vi "Test Joystick.vi"() -> ()   [LabVIEW 2018]
uses:
  <vilib>/Instr/_visa.llb/VISA Configure Serial Port (Instr).vi
panel:
  in  "TITL":bool
  in  "PAN":bool
  out "pan":dbl
  out "tilt angle":dbl format="%.2f"
  in  "autoFocus":bool
  out "Cam rcv":string
  in  "Clear":bool
  in  "Menu":bool caption="Open"
  in  "Aux":bool caption="Open"
  in  "Tele":bool caption="Open"
  in  "wide":bool caption="Wide"
  in  "OFF":bool caption="Open"
  in  "ON":bool caption="Open"
  in  "Near":bool caption="Open"
  in  "Far":bool
  in  "ACK":bool caption="Open"
  in  "Shot":bool caption="Open"
  in  "Open":bool
  in  "Close":bool
  out "Keypad sent":string
  in  "VISA resource name 2":refnum<visa-resource-name>
  in  "Stop Button":bool
  in  "VISA resource name":refnum<visa-resource-name>
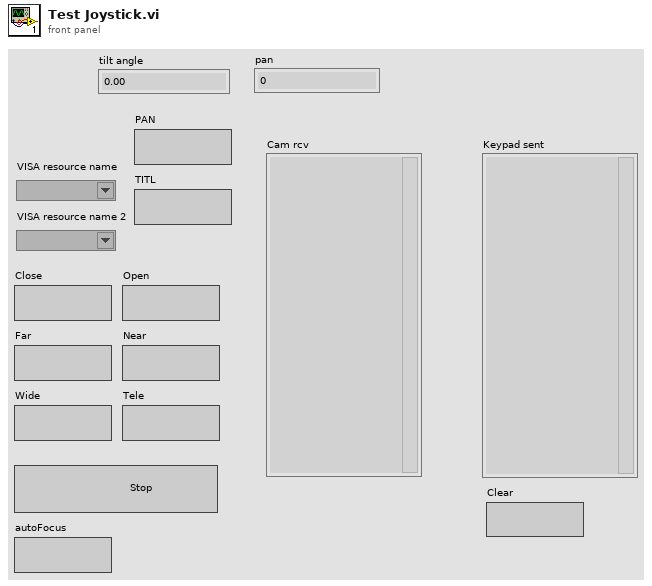
[diagram p1: front panel]
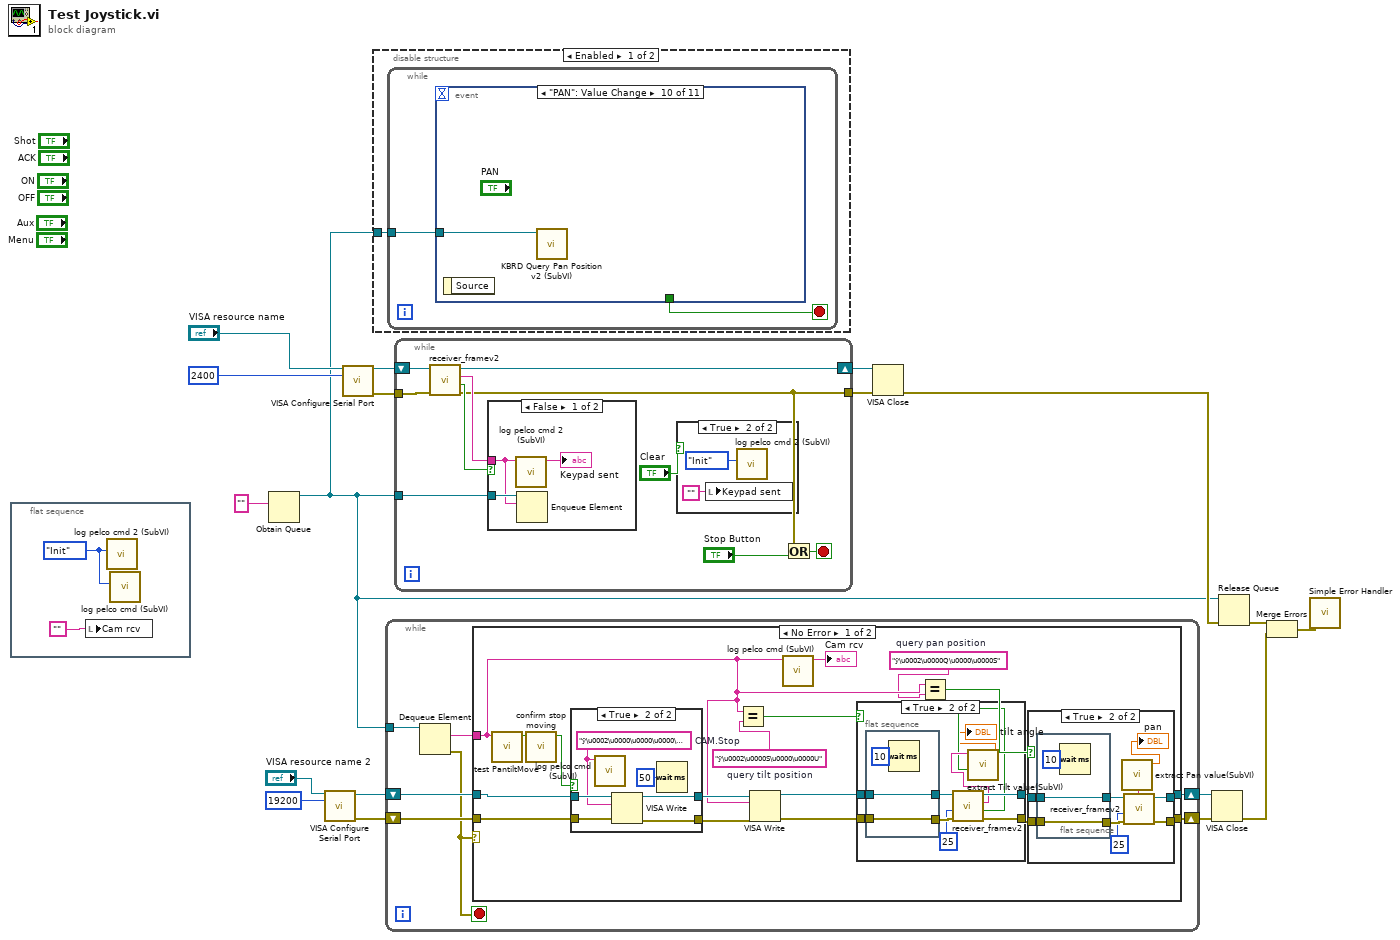
[diagram p0: block diagram]
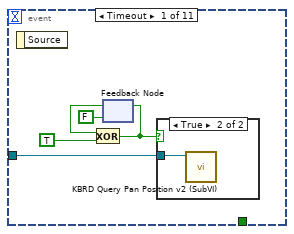
[diagram p2: hidden frame]
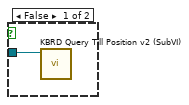
[diagram p3: hidden frame]
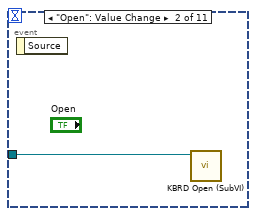
[diagram p4: hidden frame]
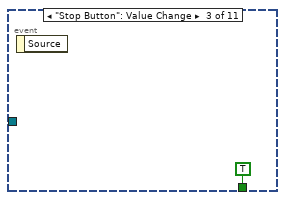
[diagram p5: hidden frame]
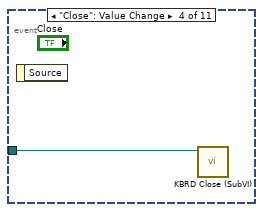
[diagram p6: hidden frame]
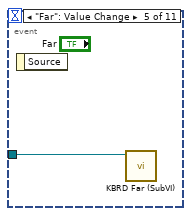
[diagram p7: hidden frame]
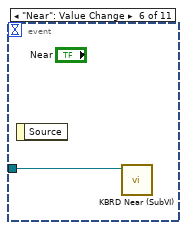
[diagram p8: hidden frame]
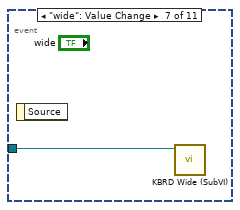
[diagram p9: hidden frame]
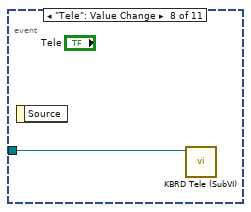
[diagram p10: hidden frame]
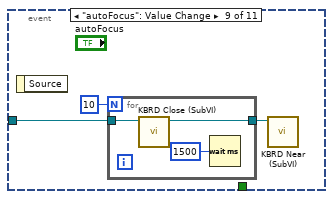
[diagram p11: hidden frame]
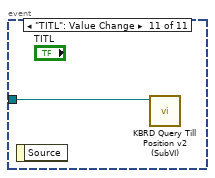
[diagram p12: hidden frame]
diagram:
  n1 = flat-sequence {
    frame #0 {
      w20 = enum16{"Log", "Init"}."Init" ("Enum(log)")
      n2 = local write "Cam rcv"("") -> ()
      n3 = call "log pelco cmd 2 (SubVI).vi"("Enum(log)"=w20) -> ()  [unwired: 10 in, 1 out]
      n4 = call "log pelco cmd (SubVI).vi"("Enum(log)"=w20) -> ()  [unwired: 10 in, 1 out]
    }
  }
  n5 = Obtain Queue(element data type="") -> (queue out=w1:refnum<queue>)  [unwired: 4 in, 2 out]
  n6 = call-poly "VISA Configure Serial Port"("VISA resource name"="VISA resource name 2", "baud rate (9600)"=u32 19200) -> ("VISA resource name out"=w9:refnum<visa-resource-name>, "error out"=w8:errorcluster)  [unwired: 12 in]
  n7 = call-poly "VISA Configure Serial Port"("VISA resource name"="VISA resource name", "baud rate (9600)"=u32 2400) -> ("VISA resource name out"=w16:refnum<visa-resource-name>, "error out"=w15:errorcluster)  [unwired: 12 in]
  n8 = disable-structure shown="Enabled" {
    disable-tunnel: w1 -> [w21 _]
    frame Enabled {
      n9 = while {
        tunnel: w21 -> [w23]
        stop <- w22 stop-if-true
        n10 = event shown="[9] \"PAN\": Value Change" {
          selector: _ -> [_ _ _ _ _ _ _ _ _ _ _]
          dyn-events: _ -> [_ _ _ _ _ _ _ _ _ _ _]
          timeout: _ -> [_ _ _ _ _ _ _ _ _ _ _]
          tunnel: w23 -> [w24 w31 _ w33 w34 w35 w36 w37 w39 w44 w45]
          tunnel: [_ _ TRUE _ _ _ _ _ _ _ _] -> w22
          event Timeout {
            n11 = event-data() -> ()  [unwired: 1 in, 1 out]
            n12 = feedback #1(FALSE) -> (w27:bool)
            n13 = Exclusive Or(1:TRUE, 2:w27) -> (0:w26:bool)
            n14 = feedback-in #1(w26) -> ()
            n15 = case shown="True" w26 {
              tunnel: w24 -> [w29 w30]
              frame False {
                n16 = call "KBRD Query Till Position v2 (SubVI).vi"("Queue in"=w29) -> ()  [unwired: 10 in, 1 out]
              }
              frame True {
                n17 = call "KBRD Query Pan Position v2 (SubVI).vi"("Queue in"=w30) -> ()  [unwired: 10 in, 1 out]
              }
            }
          }
          event "Open": Value Change {
            n18 = event-data() -> ()  [unwired: 1 in, 1 out]
            n19 = call "KBRD Open (SubVI).vi"("Queue in"=w31) -> ()  [unwired: 11 in]
          }
          event "Stop Button": Value Change {
            n20 = event-data() -> ()  [unwired: 1 in, 1 out]
          }
          event "Close": Value Change {
            n21 = event-data() -> ()  [unwired: 1 in, 1 out]
            n22 = call "KBRD Close (SubVI).vi"("Queue in"=w33) -> ()  [unwired: 10 in, 1 out]
          }
          event "Far": Value Change {
            n23 = event-data() -> ()  [unwired: 1 in, 1 out]
            n24 = call "KBRD Far (SubVI).vi"("Queue in"=w34) -> ()  [unwired: 11 in]
          }
          event "Near": Value Change {
            n25 = event-data() -> ()  [unwired: 1 in, 1 out]
            n26 = call "KBRD Near (SubVI).vi"("Queue in"=w35) -> ()  [unwired: 11 in]
          }
          event "wide": Value Change {
            n27 = event-data() -> ()  [unwired: 1 in, 1 out]
            n28 = call "KBRD Wide (SubVI).vi"("Queue in"=w36) -> ()  [unwired: 11 in]
          }
          event "Tele": Value Change {
            n29 = event-data() -> ()  [unwired: 1 in, 1 out]
            n30 = call "KBRD Tele (SubVI).vi"("Queue in"=w37) -> ()  [unwired: 11 in]
          }
          event "autoFocus": Value Change {
            n31 = event-data() -> ()  [unwired: 1 in, 1 out]
            n32 = for {
              N: 10 -> [_]
              tunnel: w39 -> [w43]
              tunnel: [w42] -> w38
              n33 = call "KBRD Close (SubVI).vi"("Queue in"=w43) -> ("dup Quece"=w42:refnum<queue>)  [unwired: 10 in]
              n34 = Wait (ms)(milliseconds to wait=u32 1500) -> ()  [unwired: 1 out]
            }
            n35 = call "KBRD Near (SubVI).vi"("Queue in"=w38) -> ()  [unwired: 11 in]
          }
          event "PAN": Value Change {
            n36 = event-data() -> ()  [unwired: 1 in, 1 out]
            n37 = call "KBRD Query Pan Position v2 (SubVI).vi"("Queue in"=w44) -> ()  [unwired: 10 in, 1 out]
          }
          event "TITL": Value Change {
            n38 = event-data() -> ()  [unwired: 1 in, 1 out]
            n39 = call "KBRD Query Till Position v2 (SubVI).vi"("Queue in"=w45) -> ()  [unwired: 10 in, 1 out]
          }
        }
      }
    }
    frame Disabled {
    }
  }
  n40 = while {
    tunnel: w1 -> [w52]
    shift-right: [w49] -> w7
    shift-left: w8 -> [w50]
    shift-right: [w47] -> w6
    shift-left: w9 -> [w51]
    stop <- w46 stop-if-true
    n41 = Dequeue Element(queue=w52) -> (element=w48:string, error out=w46:errorcluster)  [unwired: 2 in, 2 out]
    n42 = case shown="No Error" w46 {
      tunnel: w51 -> [w68 w110]
      tunnel: w50 -> [w67 w109]
      tunnel: [w53 w109] -> w49
      tunnel: w48 -> [w59 _]
      tunnel: [w54 w110] -> w47
      frame No Error {
        w58 = "ÿ\u0002\u0000Q\u0000\u0000S"  # query pan position
        w63 = "ÿ\u0002\u0000S\u0000\u0000U"  # query tilt position
        n43 = call "test PantiltMove.vi"("PelcoD frame"=w59) -> ("Pantilt Move?"=w70:bool)  [unwired: 10 in]
        n44 = call "confirm stop moving.vi"("moving?"=w70) -> ("Boolean"=w69:bool)  [unwired: 10 in]
        n45 = case shown="True" w69 {
          tunnel: w68 -> [w102 w108]
          tunnel: w67 -> [w101 w107]
          tunnel: [w101 w106] -> w66
          tunnel: [w102 w105] -> w65
          frame False {
          }
          frame True {
            w104 = "ÿ\u0002\u0000\u0000\u0000\u0000\u0002"  # CAM.Stop
            n46 = call "log pelco cmd (SubVI).vi"("String"=w104) -> ()  [unwired: 10 in, 1 out]
            n47 = VISA Write(VISA resource name=w108, write buffer=w104, error in (no error)=w107) -> (VISA resource name out=w105:refnum<visa-resource-name>, error out=w106:errorcluster)  [unwired: 1 out]
            n48 = Wait (ms)(milliseconds to wait=u32 50) -> ()  [unwired: 1 out]
          }
        }
        n49 = Equal?(x=w59, y=w63) -> (x = y?=w62:bool)
        n50 = VISA Write(VISA resource name=w65, write buffer=w59, error in (no error)=w66) -> (VISA resource name out=w61:refnum<visa-resource-name>, error out=w60:errorcluster)  [unwired: 1 out]
        n51 = call "log pelco cmd (SubVI).vi"("String"=w59) -> ("Cam rcv"=→"Cam rcv":string)  [unwired: 10 in]
        n52 = case shown="True" w62 {
          tunnel: w61 -> [w87 w97]
          tunnel: w60 -> [w86 w96]
          tunnel: [w87 w93] -> w56
          tunnel: [w86 w92] -> w55
          frame False {
          }
          frame True {
            n53 = flat-sequence {
              tunnel: [w99] -> w94
              tunnel: w97 -> [w99]
              tunnel: [w98] -> w95
              tunnel: w96 -> [w98]
              frame #0 {
                n54 = Wait (ms)(milliseconds to wait=u32 10) -> ()  [unwired: 1 out]
              }
            }
            n55 = call "receiver_framev2.vi"("error in (no error)"=w95, "Timeout(100ms)"=u32 25, "Visa In"=w94) -> ("error out"=w92:errorcluster, "TimeOut?"=w89:bool, "response"=w90:string, "Visa out"=w93:refnum<visa-resource-name>)  [unwired: 5 in]
            n56 = call "extract Tilt value(SubVI).vi"("Time out?"=w89, "Pelco-D response"=w90) -> ("tilt1"=→"tilt angle":dbl)  [unwired: 8 in, 1 out]
          }
        }
        n57 = Equal?(x=w59, y=w58) -> (x = y?=w57:bool)
        n58 = case shown="True" w57 {
          tunnel: w56 -> [w72 w82]
          tunnel: w55 -> [w71 w81]
          tunnel: [w72 w78] -> w54
          tunnel: [w71 w77] -> w53
          frame False {
          }
          frame True {
            n59 = flat-sequence {
              tunnel: [w84] -> w79
              tunnel: w82 -> [w84]
              tunnel: [w83] -> w80
              tunnel: w81 -> [w83]
              frame #0 {
                n60 = Wait (ms)(milliseconds to wait=u32 10) -> ()  [unwired: 1 out]
              }
            }
            n61 = call "receiver_framev2.vi"("error in (no error)"=w80, "Timeout(100ms)"=u32 25, "Visa In"=w79) -> ("error out"=w77:errorcluster, "TimeOut?"=w73:bool, "response"=w74:string, "Visa out"=w78:refnum<visa-resource-name>)  [unwired: 5 in]
            n62 = call "extract Pan value(SubVI).vi"("TimeOut"=w73, "response"=w74) -> ("pan angle"=→"pan":dbl)  [unwired: 8 in, 1 out]
          }
        }
      }
      frame Error {
      }
    }
  }
  n63 = while {
    tunnel: w15 -> [w119]
    shift-right: [w118] -> w14
    shift-left: w16 -> [w120]
    tunnel: [w113] -> w13
    tunnel: w1 -> [w112]
    stop <- w114 stop-if-true
    n64 = call "receiver_framev2.vi"("error in (no error)"=w119, "Visa In"=w120) -> ("error out"=w113:errorcluster, "TimeOut?"=w117:bool, "response"=w116:string, "Visa out"=w118:refnum<visa-resource-name>)  [unwired: 6 in]
    n65 = case shown="False" w117 {
      tunnel: w116 -> [w124 _]
      tunnel: w112 -> [w125 _]
      frame False {
        n66 = call "log pelco cmd 2 (SubVI).vi"("String"=w124) -> ("Cam rcv"=→"Keypad sent":string)  [unwired: 10 in]
        n67 = Enqueue Element(queue=w125, element=w124) -> ()  [unwired: 2 in, 3 out]
      }
      frame True {
      }
    }
    n68 = case shown="True" "Clear" {
      frame False {
      }
      frame True {
        n69 = local write "Keypad sent"("") -> ()
        n70 = call "log pelco cmd 2 (SubVI).vi"("Enum(log)"=enum16{"Log", "Init"}."Init") -> ()  [unwired: 10 in, 1 out]
      }
    }
    n71 = Or(x=w113, y="Stop Button") -> (x .or. y?=w114:bool)
  }
  n72 = VISA Close(VISA resource name=w14, error in (no error)=w13) -> (error out=w5:errorcluster)
  n73 = VISA Close(VISA resource name=w6, error in (no error)=w7) -> (error out=w3:errorcluster)
  n74 = Release Queue(queue=w1, error in (no error)=w5) -> (error out=w4:errorcluster)  [unwired: 1 in, 2 out]
  n75 = Merge Errors(w4, w3) -> (w2:errorcluster)
  n76 = call <vilib>:"Simple Error Handler.vi"("error in (no error)"=w2) -> ()  [unwired: 4 in, 5 out]
